vi "Assert Equal Value_Variant.vi"(4 "Execution time (s)":dbl=-1.0, 5 "Assert Only? (F)":bool, 6 "error code (1)":i32=1, 7 "Label":string, 8 "error in (no error)":errorcluster, 10 "Y":variant, 11 "X":variant) -> (0 "error out":errorcluster)   [LabVIEW 2013, in "Caraya.lvlib" / "Assert.lvclass"]
doc: "Generates an error if the input condition is not met.\n\nThis method compares the value of the inputs, irrespective of the type representation.\nAsserts TRUE if input values are equal.\nAsserts FALSE otherwise.\n\nex: Two integer inputs of equal value but of different type representation (U8 and I32) will assert TRUE."
uses:
  Assert.lvclass
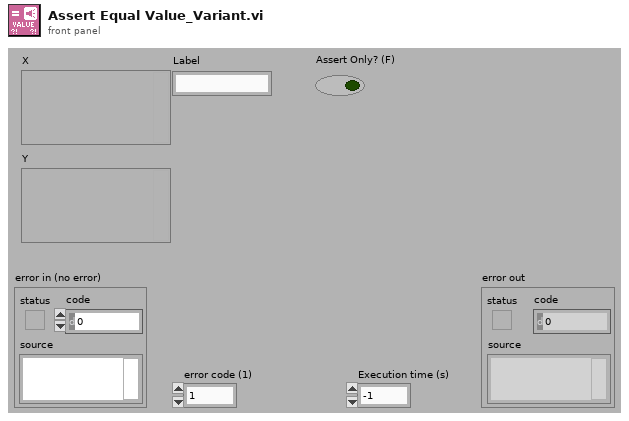
[diagram p1: front panel]
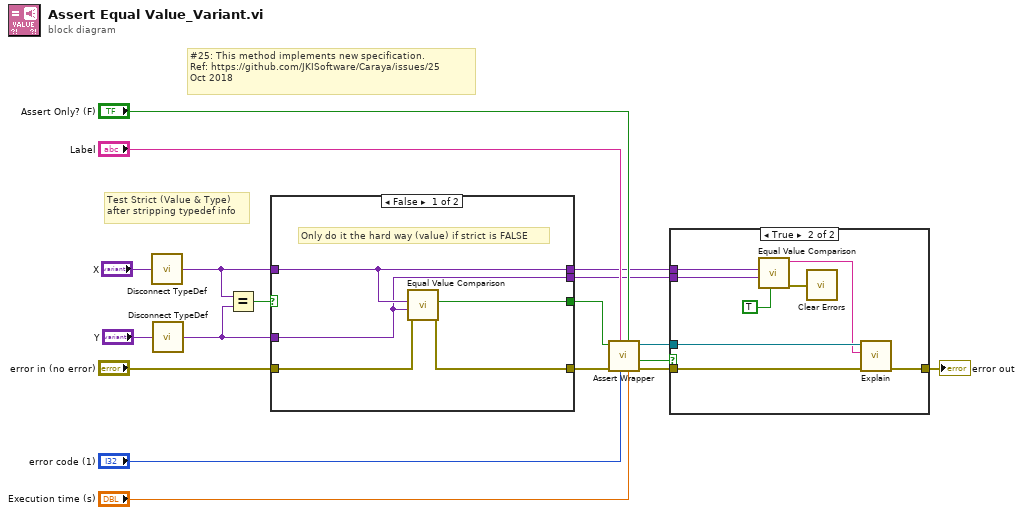
[diagram p0: block diagram]
diagram:
  # "Test Strict (Value & Type)\nafter stripping typedef info"
  # "#25: This method implements new specification.\nRef: https://github.com/JKISoftware/Caraya/issues/25\nOct 2018"
  n1 = call "Disconnect TypeDef.vi"("Variant"="X") -> ("Variant Out"=w12:variant)
  n2 = call "Disconnect TypeDef.vi"("Variant"="Y") -> ("Variant Out"=w10:variant)
  n3 = Equal?(x=w12, y=w10) -> (x = y?=w14:bool)
  n4 = case shown="False" w14 {
    selector: w14 -> [_ w27]
    tunnel: [w23 w27] -> w15
    tunnel: "error in (no error)" -> [w22 w26]
    tunnel: [w21 w26] -> w8
    tunnel: w12 -> [w20 w25]
    tunnel: w10 -> [w19 w24]
    tunnel: [w20 w25] -> w4
    tunnel: [w19 w24] -> w3
    frame False {
      # "Only do it the hard way (value) if strict is FALSE"
      n5 = call "Equal Value Comparison.vi"("error in (no error)"=w22, "Y"=w19, "X"=w20) -> ("error out"=w21:errorcluster, "Equal Values?"=w23:bool)  [unwired: 6 in, 1 out]
    }
    frame True {
    }
  }
  n6 = call "Assert Wrapper.vi"("Execution time (s)"="Execution time (s)", "Assert Only? (F)"="Assert Only? (F)", "error code (1)"="error code (1)", "Label"="Label", "error in (no error)"=w8, "Assert?"=w15) -> ("error out"=w7:errorcluster, "Verbose"=w2:bool, "Assert out"=w1:refnum<class "Assert.lvclass">)  [unwired: 3 in]
  n7 = case shown="True" w2 {
    tunnel: [w28 w36] -> w5
    tunnel: w1 -> [_ w35]
    tunnel: w7 -> [w28 w34]
    tunnel: w4 -> [_ w32]
    tunnel: w3 -> [_ w31]
    frame False {
    }
    frame True {
      n8 = call "Equal Value Comparison.vi"("verbose? (F)"=TRUE, "Y"=w31, "X"=w32) -> ("error out"=w29:errorcluster, "Verbose output"=w33:string)  [unwired: 6 in, 1 out]
      n9 = call <vilib>:"Clear Errors.vi"("error in (no error)"=w29) -> ()  [unwired: 6 in, 1 out]
      n10 = call-dynamic "Explain.vi"("error in (no error)"=w34, "Verbose Explanation"=w33, "Assert in"=w35) -> ("error out"=w36:errorcluster)  [unwired: 7 in, 1 out]
    }
  }
  "error out" <- w5
